vi "Clear Audio Backend.vi"(8 "error in (no error)":errorcluster) -> (0 "error out":errorcluster)   [LabVIEW 2020, in "G-Audio.lvlib"]
doc: "Clears the audio backend. Will automatically stop and clear all audio devices."
uses:
  G-Audio.lvlib
  <vilib>/Utility/error.llb/Error Cluster From Error Code.vi
  lib/g_audio_32.dll
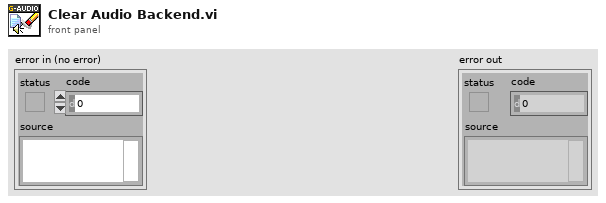
[diagram p1: front panel]
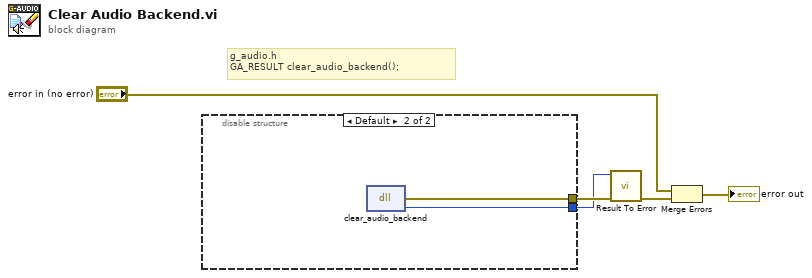
[diagram p0: block diagram]
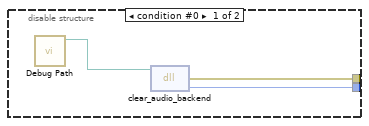
[diagram p2: hidden frame]
diagram:
  # "g_audio.h\nGA_RESULT clear_audio_backend();"
  n1 = disable-structure shown="Default" {
    disable-tunnel: [w7 w10] -> w4
    disable-tunnel: [w6 w9] -> w3
    frame condition #0 {
      n2 = call "Debug Path.vi"() -> ("Debug Path"=w8:path)  [unwired: 11 in]
      n3 = dll-call lib="?" fn="clear_audio_backend"(path in=w8) -> (error out=w7:errorcluster, "result"=w6:i32)  [unwired: 2 in, 1 out]
    }
    frame condition #1 (active) {
      n4 = dll-call lib="C:/github/dataflowg/g-audio/src/LabVIEW/G-Audio/lib/g_audio_*.*" fn="clear_audio_backend"() -> (error out=w10:errorcluster, "result"=w9:i32)  [unwired: 3 in, 1 out]
    }
  }
  n5 = call "Result To Error.vi"("error in (no error)"=w4, "Result Code"=w3) -> ("error out"=w5:errorcluster)  [unwired: 9 in]
  n6 = Merge Errors("error in (no error)", w5) -> (→"error out":errorcluster)
